vi "Prepare Scope.vi"(8 "error in":errorcluster, 9 "Channel List In":string, 10 "Fgen Session In":refnum<k15>, 11 "measurement configuration in":T2={"Resource Name(s)"=[], "Number Of Records"=2, "Timeout (s)"=5.0, "Configuration File Path"="", "Delay Mode"="On", "Horizontal Position"=0.0, "Length Unit"="Percentage", "Record Length"=100.0, "Stream To File Path"=""} {"Record Length" format="%#_6ps"; "Horizontal Position" min=0.0 max=100.0 step=5.0 format="%#_6ps"; "Timeout (s)" format="%#_6p"}) -> (0 "error out":errorcluster, 1 "Channel List Out":string, 2 "Fgen Session Out":refnum<k15>, 3 "measurement configuration out":T2={"Resource Name(s)"=[], "Number Of Records"=2, "Timeout (s)"=5.0, "Configuration File Path"="", "Delay Mode"="On", "Horizontal Position"=0.0, "Length Unit"="Percentage", "Record Length"=100.0, "Stream To File Path"=""} {"Record Length" format="%#_6ps"; "Horizontal Position" min=0.0 max=100.0 step=5.0 format="%#_6ps"; "Timeout (s)" format="%#_6p"}, 4 "Actual Settings":T1)   [LabVIEW 2025, in "Ni-Scope-Multirecords.lvclass"]
uses:
  Ni-Scope-Multirecords.lvclass
  Measurement Configuration.ctl
  <instrlib>/niScope/Configure/niScope Import Attribute Configuration File.vi
  Ni-Scope-Multirecords.lvclass/Ni-Scope-Multirecords.ctl
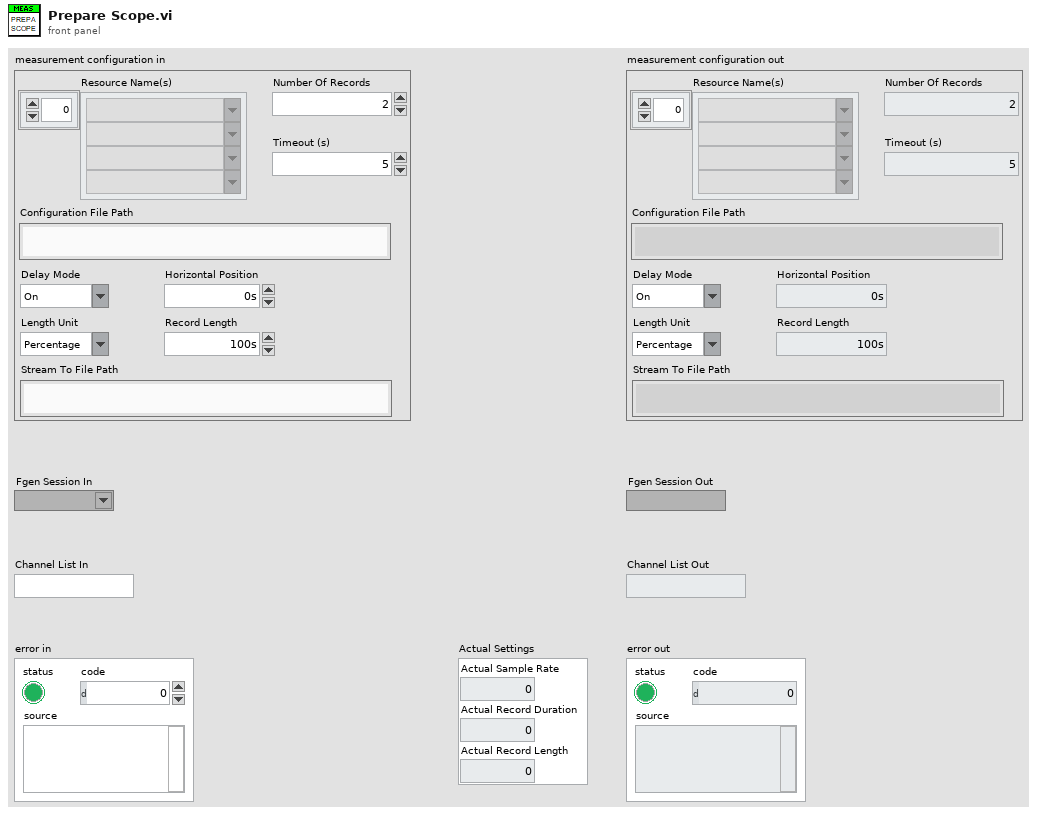
[diagram p1: front panel]
types:
  T1 = cluster{"Actual Sample Rate":dbl, "Actual Record Duration":dbl, "Actual Record Length":i32}
  T2 = typedef "Ni-Scope-Multirecords.lvclass/Measurement Configuration.ctl" = cluster{"Resource Name(s)":string[], "Number Of Records":i32, "Timeout (s)":dbl, "Configuration File Path":string, "Delay Mode":string, "Horizontal Position":dbl, "Length Unit":string, "Record Length":dbl, "Stream To File Path":string}
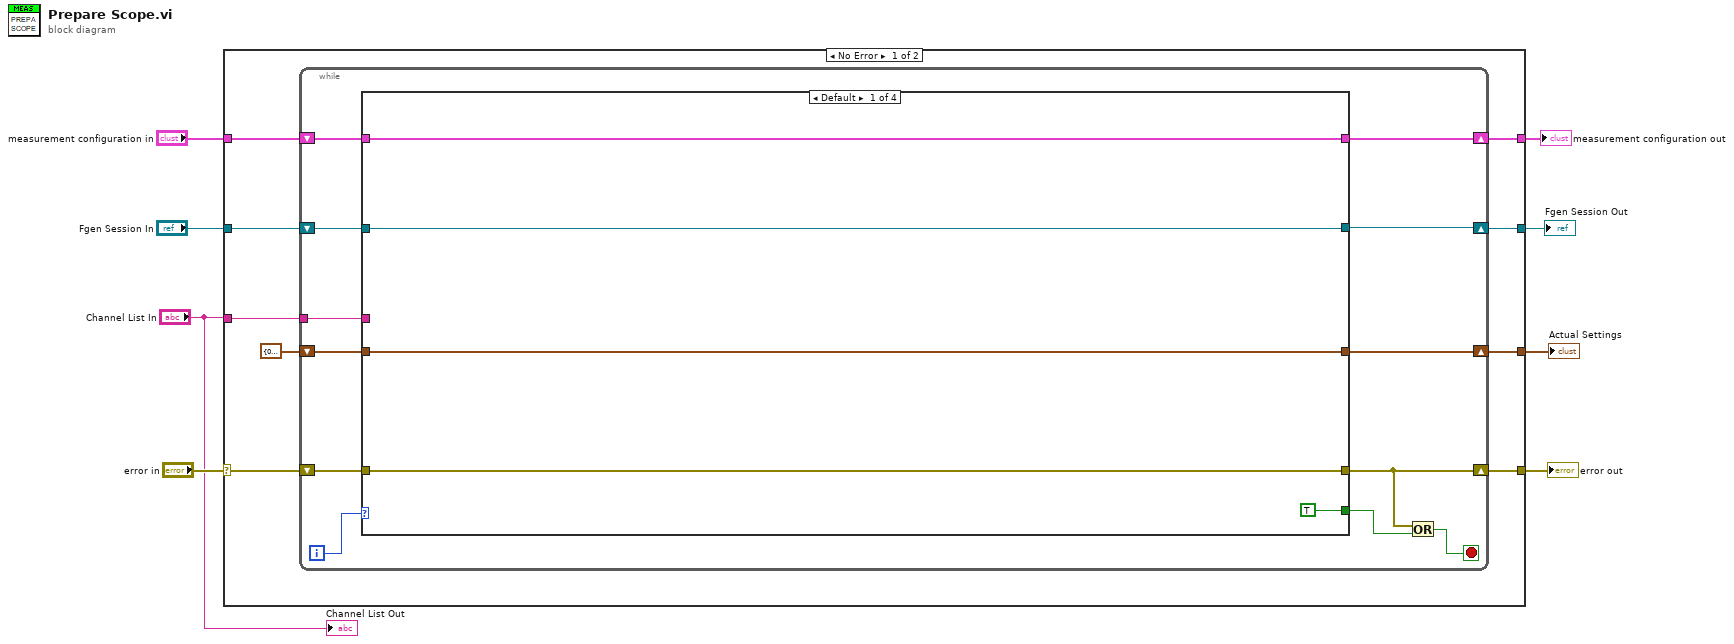
[diagram p0: block diagram]
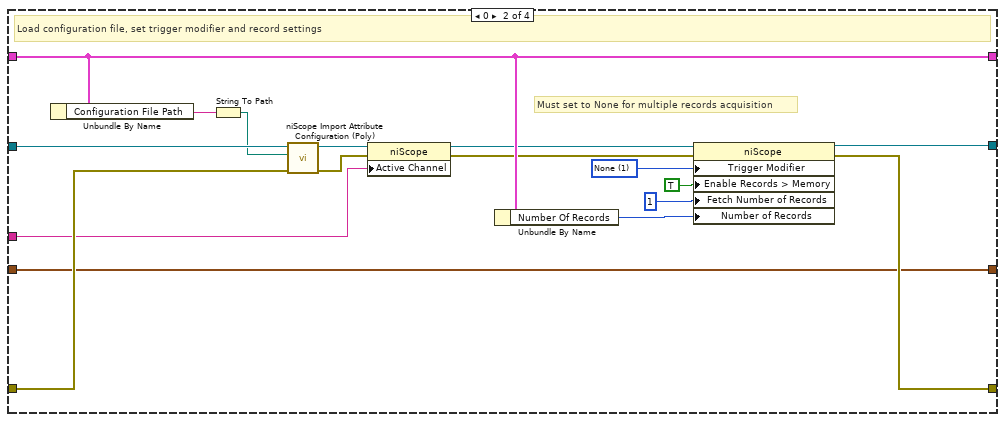
[diagram p2: hidden frame]
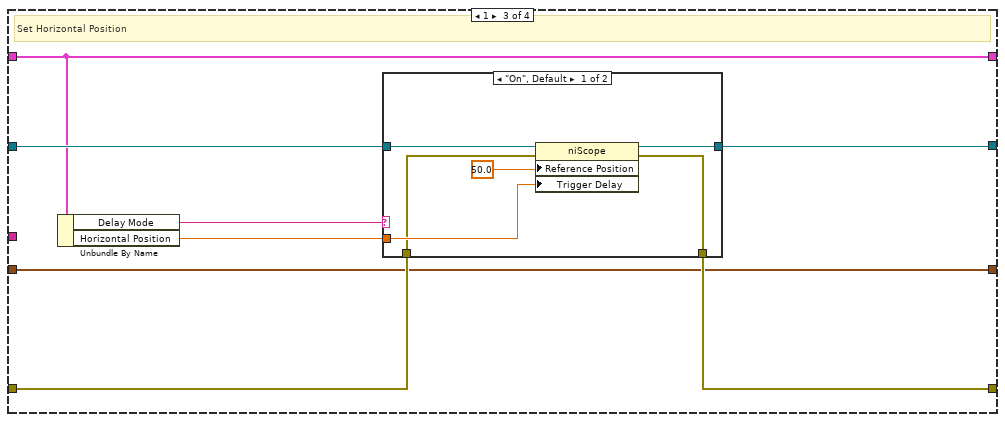
[diagram p3: hidden frame]
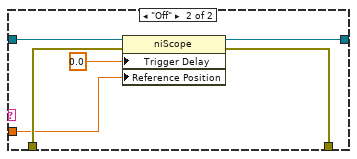
[diagram p4: hidden frame]
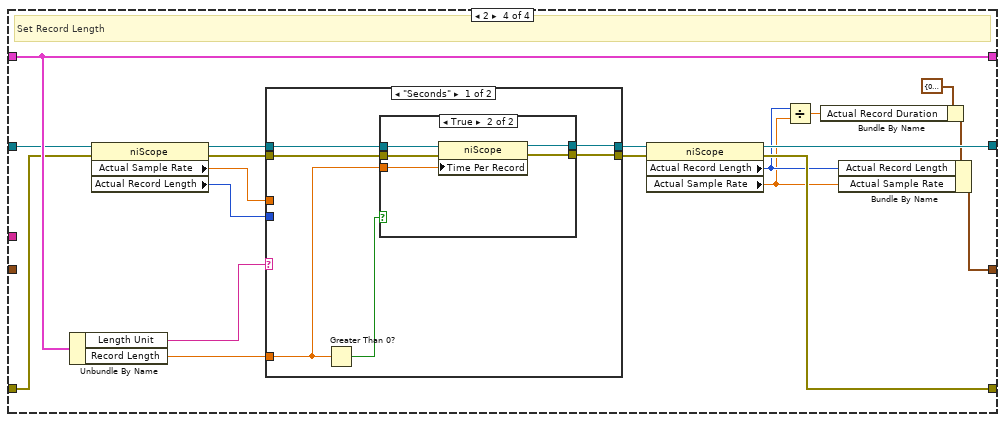
[diagram p5: hidden frame]
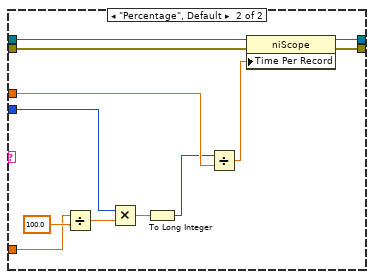
[diagram p7: hidden frame]
diagram:
  n1 = case shown="No Error" "error in" {
    selector: "error in" -> [w17 w117]
    tunnel: "measurement configuration in" -> [w16 w118]
    tunnel: [w12 w118] -> w6
    tunnel: [w11 w117] -> w5
    tunnel: "Fgen Session In" -> [w15 w116]
    tunnel: "Channel List In" -> [w14 _]
    tunnel: [w13 w116] -> w3
    tunnel: [w10 _] -> w2
    frame No Error {
      n2 = while {
        shift-right: [w25] -> w11
        shift-left: w17 -> [w28]
        shift-right: [w26] -> w12
        shift-left: w16 -> [w27]
        shift-right: [w20] -> w13
        shift-left: w15 -> [w22]
        tunnel: w14 -> [w21]
        shift-right: [w19] -> w10
        shift-left: T1 {"Actual Sample Rate"=0.0, "Actual Record Duration"=0.0, "Actual Record Length"=0} ("Actual Settings") -> [w18]
        i -> [w29]
        stop <- w23 stop-if-true
        n3 = case shown="Default" w29 {
          tunnel: w28 -> [w34 w50 w55 w86]
          tunnel: [w34 w48 w54 w87] -> w25
          tunnel: w27 -> [w33 w46 w58 w90]
          tunnel: [w33 w46 w58 w90] -> w26
          tunnel: [TRUE _ _ _] -> w24
          tunnel: w22 -> [w31 w51 w59 w85]
          tunnel: w21 -> [_ w36 _ _]
          tunnel: [w31 w49 w57 w84] -> w20
          tunnel: [w30 w35 w52 w81] -> w19
          tunnel: w18 -> [w30 w35 w52 _]
          frame Default {
          }
          frame 0 {
            w47 = 1 items=["None"=1, "Auto Trigger"=2] ("Triggering:Trigger Modifier")
            # "Must set to None for multiple records acquisition"
            # "Load configuration file, set trigger modifier and record settings"
            n4 = Unbundle By Name(w46) -> ("Configuration File Path"=w45:string)
            n5 = String To Path(string=w45) -> (path=w44:path)
            n6 = call-poly <instrlib>:"niScope Import Attribute Configuration (Poly).vi"("error in"=w50, "file path"=w44, "instrument handle"=w51) -> ("error out"=w37:errorcluster, "instrument handle out"=w39:refnum<k15>)  [unwired: 7 in]
            n7 = property class="niScope"(reference=w39, error in=w37, "Active Channel"=w36) -> (reference out=w38:refnum<k15>, error out=w40:errorcluster)
            n8 = Unbundle By Name(w46) -> ("Number Of Records"=w41:i32)
            n9 = property class="niScope"(reference=w38, error in=w40, "Trigger Modifier"=w47, "Enable Records > Memory"=TRUE ("Horizontal:Enable Records > Memory"), "Fetch Number of Records"=1 ("Fetch:Fetch Number of Records"), "Number of Records"=w41) -> (reference out=w49:refnum<k15>, error out=w48:errorcluster)
          }
          frame 1 {
            # "Set Horizontal Position"
            n10 = Unbundle By Name(w58) -> ("Delay Mode"=w53:string, "Horizontal Position"=w56:dbl)
            n11 = case shown="\"On\", Default" w53 {
              tunnel: w59 -> [w65 w71]
              tunnel: [w64 w70] -> w57
              tunnel: w56 -> [w62 w66]
              tunnel: w55 -> [w61 w69]
              tunnel: [w60 w68] -> w54
              frame "On", Default {
                n12 = property class="niScope"(reference=w65, error in=w61, "Reference Position"=50.0 ("Horizontal:Reference Position"), "Trigger Delay"=w62) -> (reference out=w64:refnum<k15>, error out=w60:errorcluster)
              }
              frame "Off" {
                n13 = property class="niScope"(reference=w71, error in=w69, "Trigger Delay"=0.0 ("Triggering:Trigger Delay"), "Reference Position"=w66) -> (reference out=w70:refnum<k15>, error out=w68:errorcluster)
              }
            }
          }
          frame 2 {
            # "Set Record Length"
            n14 = Unbundle By Name(w90) -> ("Length Unit"=w89:string, "Record Length"=w88:dbl)
            n15 = property class="niScope"(reference=w85, error in=w86) -> (reference out=w74:refnum<k15>, error out=w75:errorcluster, "Actual Sample Rate"=w83:dbl, "Actual Record Length"=w76:i32)
            n16 = case shown="\"Seconds\"" w89 {
              tunnel: w76 -> [_ w115]
              tunnel: w83 -> [_ w111]
              tunnel: w88 -> [w91 w109]
              tunnel: w75 -> [w94 w106]
              tunnel: w74 -> [w95 w107]
              tunnel: [w92 w105] -> w73
              tunnel: [w93 w104] -> w72
              frame "Seconds" {
                n17 = Greater Than 0?(x=w91) -> (x > 0?=w96:bool)
                n18 = case shown="True" w96 {
                  tunnel: w95 -> [w98 w103]
                  tunnel: w94 -> [w97 w102]
                  tunnel: [w98 w101] -> w93
                  tunnel: [w97 w100] -> w92
                  tunnel: w91 -> [_ w99]
                  frame False {
                  }
                  frame True {
                    n19 = property class="niScope"(reference=w103, error in=w102, "Time Per Record"=w99) -> (reference out=w101:refnum<k15>, error out=w100:errorcluster)
                  }
                }
              }
              frame "Percentage", Default {
                n20 = Divide(x=w109, y=100.0) -> (x/y=w112:dbl)
                n21 = Multiply(x=w115, y=w112) -> (x*y=w114:dbl)
                n22 = To Long Integer(number=w114) -> (32bit integer=w110:i32)
                n23 = Divide(x=w110, y=w111) -> (x/y=w108:dbl)
                n24 = property class="niScope"(reference=w107, error in=w106, "Time Per Record"=w108) -> (reference out=w104:refnum<k15>, error out=w105:errorcluster)
              }
            }
            n25 = property class="niScope"(reference=w72, error in=w73) -> (reference out=w84:refnum<k15>, error out=w87:errorcluster, "Actual Record Length"=w80:i32, "Actual Sample Rate"=w79:dbl)
            n26 = Divide(x=w80, y=w79) -> (x/y=w77:dbl)
            n27 = Bundle By Name(cluster=T1 {"Actual Sample Rate"=0.0, "Actual Record Duration"=0.0, "Actual Record Length"=0} ("Actual Settings"), "Actual Record Duration"=w77) -> (w78:T1)
            n28 = Bundle By Name(cluster=w78, "Actual Record Length"=w80, "Actual Sample Rate"=w79) -> (w81:T1)
          }
        }
        n29 = Or(x=w25, y=w24) -> (x .or. y?=w23:bool)
      }
    }
    frame Error {
    }
  }
  "measurement configuration out" <- w6
  "error out" <- w5
  "Fgen Session Out" <- w3
  "Actual Settings" <- w2
  "Channel List Out" <- "Channel List In"
